vi "CarMoveTest.vi"() -> ()   [LabVIEW 2019]
uses:
  <vilib>/Utility/miscctls.llb/LVPositionTypeDef.ctl
panel:
  out "Boolean":bool
  in  "Button":bool
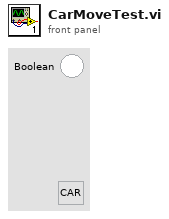
[diagram p1: front panel]
types:
  T1 = typedef "LVPositionTypeDef.ctl" = cluster{"Left":i32, "Top":i32}
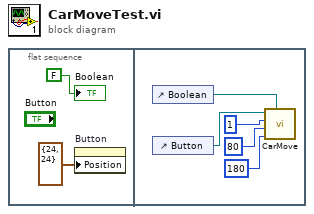
[diagram p0: block diagram]
diagram:
  n1 = flat-sequence {
    frame #0 {
      n2 = property on="Button" class="Bool"("Position"=T1 {"Left"=24, "Top"=24}) -> ()  [unwired: 2 in, 2 out]
      "Boolean" <- FALSE ("Boolean")
    }
    frame #1 {
      n3 = control-ref of="Boolean"() -> (w7:refnum<vi>)
      n4 = control-ref of="Button"() -> (w6:refnum<vi>)
      n5 = call "CarMove.vi"("X done?"=w7, "X+Y"=180, "X"=80, "speed"=u32 1, "Boolean in"=w6) -> ()  [unwired: 7 in]
    }
  }
